vi "CreateProperties.vi"(8 "error in (no error)":errorcluster, 11 "GenLVOOP in":refnum<class "GenLVOOP.lvclass">) -> (0 "error out":errorcluster, 3 "GenLVOOP out":refnum<class "GenLVOOP.lvclass">)   [LabVIEW 2013, in "GenLVOOP.lvclass"]
uses:
  GenLVOOP.lvclass
  baseClass/baseClass.lvclass
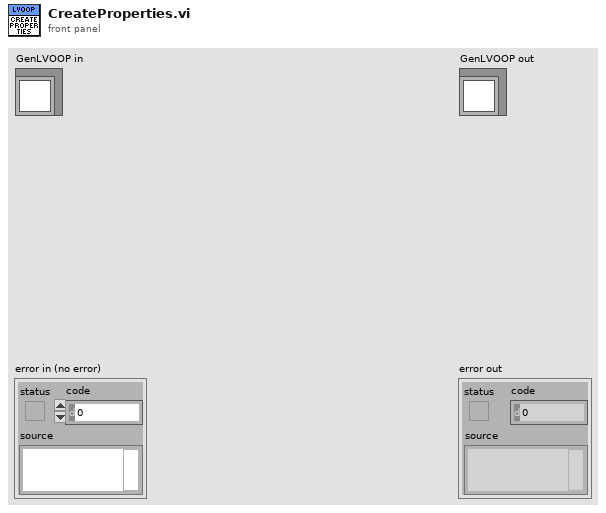
[diagram p1: front panel]
types:
  T1 = enum32{"Invalid", "Standard", "Closed", "Hidden", "Minimized", "Maximized"}
  T2 = typedef "baseClass.lvclass/propertyDef.ctl" = cluster{"Name":string, "types":T3, "UserDefined":string, "Array":bool}
  T3 = typedef "baseClass.lvclass/types.ctl" = enum16{"string", "int", "decimal", "bool", "class", "enum"}
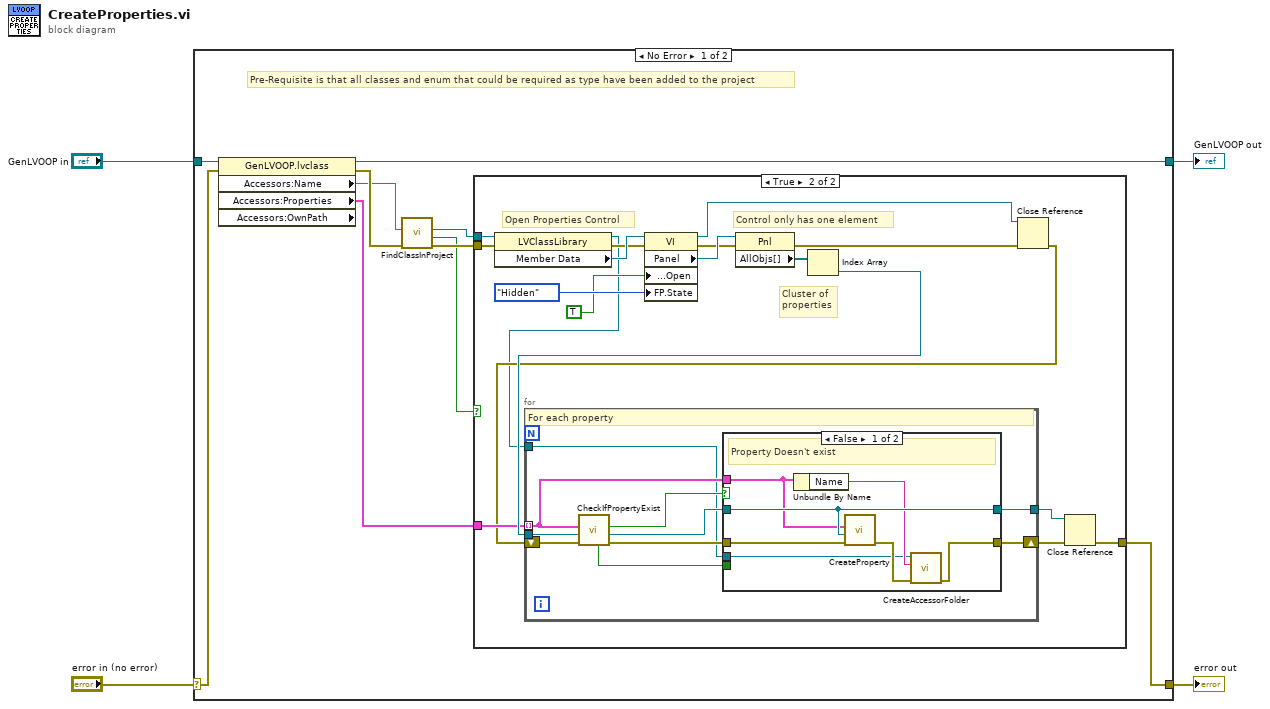
[diagram p0: block diagram]
diagram:
  n1 = case shown="No Error" "error in (no error)" {
    selector: "error in (no error)" -> [w12 w61]
    tunnel: [w13 w61] -> w3
    tunnel: [w8 w60] -> w1
    tunnel: "GenLVOOP in" -> [w14 w60]
    frame No Error {
      # "Pre-Requisite is that all classes and enum that could be required as type have been added to the project"
      n2 = property class="GenLVOOP.lvclass" props=["Accessors:Name", "Accessors:Properties", "Accessors:OwnPath"](reference=w14, error in=w12) -> (reference out=w8:refnum<class "GenLVOOP.lvclass">, error out=w10:errorcluster, "Accessors:Name"=w6:string, "Accessors:Properties"=w7:T2[])  [unwired: 1 out]
      n3 = call "FindClassInProject.vi"("error in (no error)"=w10, "Name"=w6) -> ("error out"=w9:errorcluster, "Found"=w5:bool, "LVClassLibrary Refnum"=w11:refnum<vi>)  [unwired: 7 in]
      n4 = case shown="True" w5 {
        tunnel: [w15 w31] -> w13
        tunnel: w11 -> [_ w30]
        tunnel: w9 -> [w15 w29]
        tunnel: w7 -> [_ w27]
        frame False {
        }
        frame True {
          # "Cluster of \nproperties"
          # "Control only has one element"
          # "Open Properties Control"
          n5 = property class="LVClassLibrary"(reference=w30, error in=w29) -> (reference out=w16:refnum<vi>, error out=w23:errorcluster, "Member Data"=w26:refnum<vi>)
          n6 = property class="VI"(reference=w26, error in=w23, "Front Panel.Open"=TRUE ("Front Panel Window:Open"), "FP.State"=T1."Hidden" ("Front Panel Window:State")) -> (reference out=w19:refnum<vi>, error out=w20:errorcluster, "Panel"=w22:refnum<vi>)
          n7 = property class="Pnl"(reference=w22, error in=w20) -> (error out=w18:errorcluster, "AllObjs[]"=w21:refnum<vi>[])  [unwired: 1 out]
          n8 = Index Array(array=w21) -> (element=w28:refnum<vi>)  [unwired: 1 in]
          n9 = Close Reference(reference=w19, error in (no error)=w18) -> (error out=w17:errorcluster)
          n10 = for {
            tunnel: w27 -> [w36] mode=indexing
            tunnel: [w43] -> w33
            shift-right: [w42] -> w32
            shift-left: w17 -> [w39]
            tunnel: w28 -> [w38]
            tunnel: w16 -> [w34]
            # "For each property"
            n11 = call "CheckIfPropertyExist.vi"("error in"=w39, "ClusterOfProperties"=w38, "properties"=w36) -> ("error out"=w40:errorcluster, "ClusterOfProperties"=w37:refnum<vi>, "Exists"=w41:bool, "TypeMatches"=w35:bool)  [unwired: 5 in]
            n12 = case shown="False" w41 {
              tunnel: w37 -> [w50 w54]
              tunnel: [w50 w53] -> w43
              tunnel: [w45 w51] -> w42
              tunnel: w40 -> [w49 w52]
              tunnel: w36 -> [w48 _]
              tunnel: w35 -> [_ w55]
              tunnel: w34 -> [w44 _]
              frame False {
                # "Property Doesn't exist"
                n13 = Unbundle By Name(w48) -> ("Name"=w47:string)
                n14 = call "CreateProperty.vi"("error in"=w49, "ClusterOfProperties"=w50, "properties"=w48) -> ("error out"=w46:errorcluster)  [unwired: 8 in]
                n15 = call "CreateAccessorFolder.vi"("error in (no error)"=w46, "Name"=w47, "LabVIEW Class In"=w44) -> ("error out"=w45:errorcluster)  [unwired: 7 in, 1 out]
              }
              frame True {
                # "Property exists"
                n16 = case shown="True" w55 {
                  tunnel: w54 -> [w57 w59]
                  tunnel: [w57 w59] -> w53
                  tunnel: w52 -> [w56 w58]
                  tunnel: [w56 w58] -> w51
                  frame False {
                    # "#TODO \nimplement when\ntype doesnt match"
                    # "Type doesnt match"
                  }
                  frame True {
                    # "do nothing"
                    # "type matches"
                  }
                }
              }
            }
          }
          n17 = Close Reference(reference=w33, error in (no error)=w32) -> (error out=w31:errorcluster)
        }
      }
    }
    frame Error {
    }
  }
  "error out" <- w3
  "GenLVOOP out" <- w1
